vi "Divideby10FreqDivider.vi"() -> ()   [LabVIEW 2017]
uses:
  <vilib>/DAQmx/create/channels.llb/DAQmx Create Channel (CO-Pulse Generation-Ticks).vi
  <vilib>/DAQmx/configure/timing.llb/DAQmx Timing (Implicit).vi
  <resource>/objmgr/daqmx.rc
panel:
  in  "CO.Pulse.Term":tag="/Dev6/PFI12"
  in  "source of ticks":tag="/Dev6/PFI15"
  in  "counter":tag="Dev6/ctr0"
  in  "stop":bool
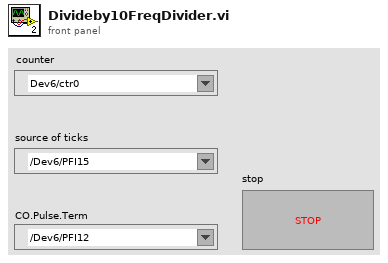
[diagram p1: front panel]
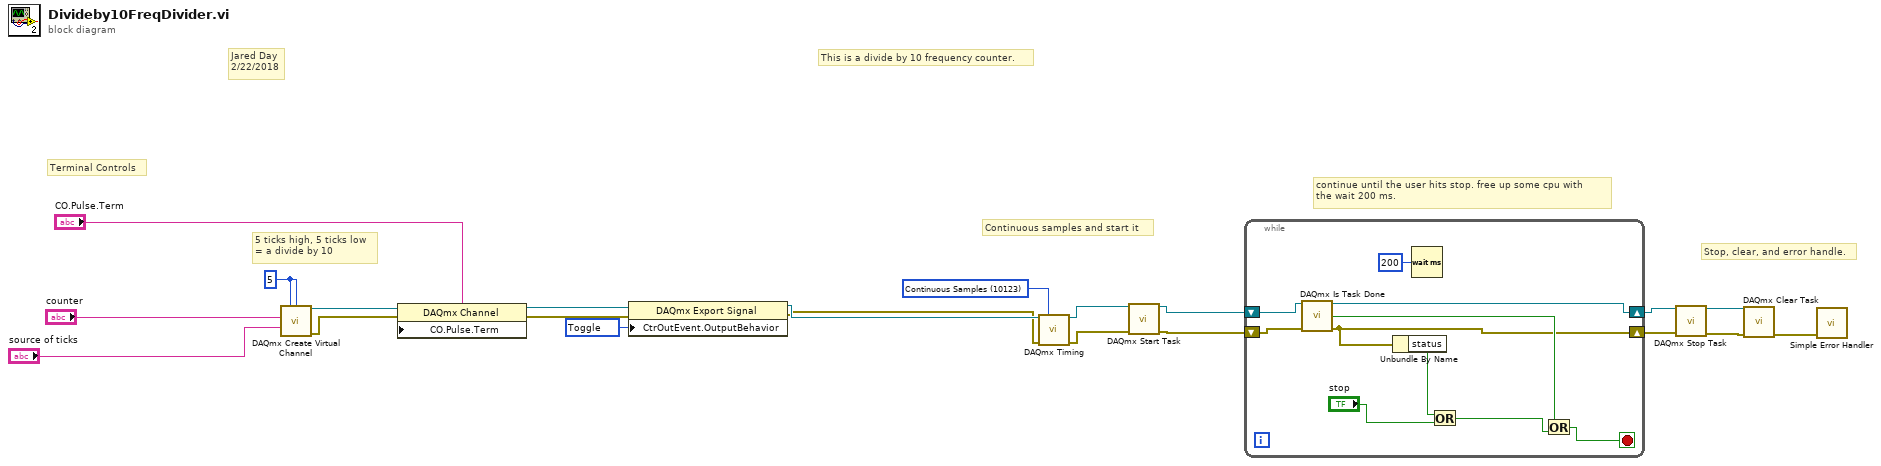
[diagram p0: block diagram]
diagram:
  w1 = 10307 items=["Pulse"=10265, "Toggle"=10307] ("CtrOutEvent.OutputBehavior")
  w16 = u32 5 ("low ticks")
  w19 = 10123 items=["Finite Samples"=10178, "Continuous Samples"=10123, "Hardware Timed Single Point"=12522] ("sample mode")
  # "Stop, clear, and error handle."
  # "continue until the user hits stop. free up some cpu with \nthe wait 200 ms."
  # "Continuous samples and start it"
  # "5 ticks high, 5 ticks low\n= a divide by 10"
  # "Terminal Controls"
  # "This is a divide by 10 frequency counter."
  # "Jared Day\n2/22/2018"
  n1 = call-poly <vilib>:"DAQmx Create Virtual Channel.vi"("high ticks"=w16, "low ticks"=w16, "counter"="counter", "source of ticks"="source of ticks") -> ("task out"=w8:refnum<k21>, "error out"=w7:errorcluster)  [unwired: 10 in]
  n2 = property class="DAQmx Channel"(reference=w8, error in=w7, "CO.Pulse.Term"="CO.Pulse.Term") -> (reference out=w5:refnum<k21>, error out=w4:errorcluster)
  n3 = property class="DAQmx Export Signal"(reference=w5, error in=w4, "CtrOutEvent.OutputBehavior"=w1) -> (reference out=w3:refnum<k21>, error out=w2:errorcluster)
  n4 = call-poly <vilib>:"DAQmx Timing.vi"("task/channels in"=w3, "sample mode"=w19, "error in"=w2) -> ("task out"=w18:refnum<k21>, "error out"=w17:errorcluster)  [unwired: 11 in]
  n5 = call <vilib>:"DAQmx Start Task.vi"("task/channels in"=w18, "error in"=w17) -> ("task out"=w15:refnum<k21>, "error out"=w14:errorcluster)  [unwired: 12 in]
  n6 = while {
    shift-right: [w24] -> w10
    shift-left: w15 -> [w30]
    shift-right: [w23] -> w11
    shift-left: w14 -> [w31]
    stop <- w25 stop-if-true
    n7 = call <vilib>:"DAQmx Is Task Done.vi"("task/channels in"=w30, "error in"=w31) -> ("task out"=w24:refnum<k21>, "task done?"=w26:bool, "error out"=w23:errorcluster)  [unwired: 11 in]
    n8 = Unbundle By Name(w23) -> ("status"=w28:bool)
    n9 = Wait (ms)(milliseconds to wait=u32 200) -> ()  [unwired: 1 out]
    n10 = Or(x=w28, y="stop") -> (x .or. y?=w27:bool)
    n11 = Or(x=w26, y=w27) -> (x .or. y?=w25:bool)
  }
  n12 = call <vilib>:"DAQmx Stop Task.vi"("task/channels in"=w10, "error in"=w11) -> ("task out"=w9:refnum<k21>, "error out"=w12:errorcluster)  [unwired: 12 in]
  n13 = call <vilib>:"DAQmx Clear Task.vi"("task in"=w9, "error in"=w12) -> ("error out"=w13:errorcluster)  [unwired: 13 in]
  n14 = call <vilib>:"Simple Error Handler.vi"("error in (no error)"=w13) -> ()  [unwired: 4 in, 5 out]
